vi "DAE Simple Pendulum Simulation.vi"() -> ()   [LabVIEW 2023]
doc: "This example demonstrates how to use the <B>DAE Radau 5th Order VI</B> to simulate the movement of a simple pendulum, which is modeled by a differential algebraic equation. In this example, the model is implemented by a cluster of formula strings and variable strings."
uses:
  <vilib>/gmath/dae.llb/Radau5_Parameters.ctl
  <vilib>/Analysis/1siggen.llb/Ramp Pattern by Samples.vi
  <vilib>/gmath/dae.llb/DAE Radau 5th Order (Formula).vi
  <vilib>/gmath/NI_DAE.lvlib
  <vilib>/gmath/NI_Gmath.lvlib
  <vilib>/Analysis/NI_AALBase.lvlib
panel:
  in  "Initial Position":dbl(slide)=0.8016949152542373 min=0.4 max=1.0 step=0.01 scale=0.4..1.0 scale format="%#_2g"
  out "pendulum":picture
  out "Simple Pendulum Simulation":picture
  # "Overview: This example demonstrates how to use the DAE Radau 5th Order VI to simulate the movement of a simple pendulum, which is modeled by a differential algebraic equation.\nRequirements: LabVIEW Full Development System\nInstructions: \n1. Run the VI.\n2. Change the Initial Position and run the VI again to see how the simple pendulum swings with different initial positions."
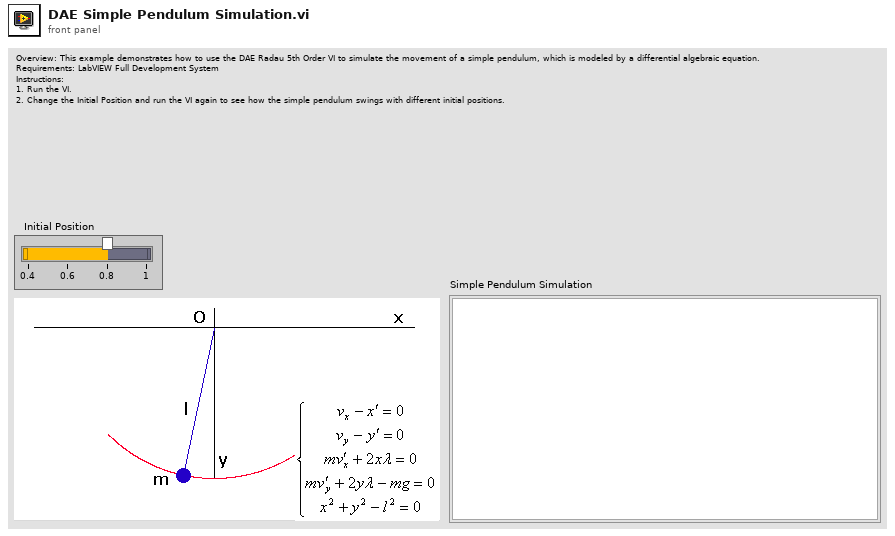
[diagram p1: front panel]
types:
  T1 = typedef "NI_DAE.lvlib/Radau5_Parameters.ctl" = cluster{"initial time":dbl, "final time":dbl, "Absolute Tolerance":dbl[], "Relative Tolerance":dbl[], "minimum time step":dbl, "maximum time step":dbl, "initial time step":dbl}
  T2 = cluster{"F(X,X',t)":string[], "X":string[], "X'":string[], "time":string}
  T3 = cluster{"Width":u16, "Style":enum32{"Solid", "Dash", "Dot", "DashDot", "DashDotDot"}}
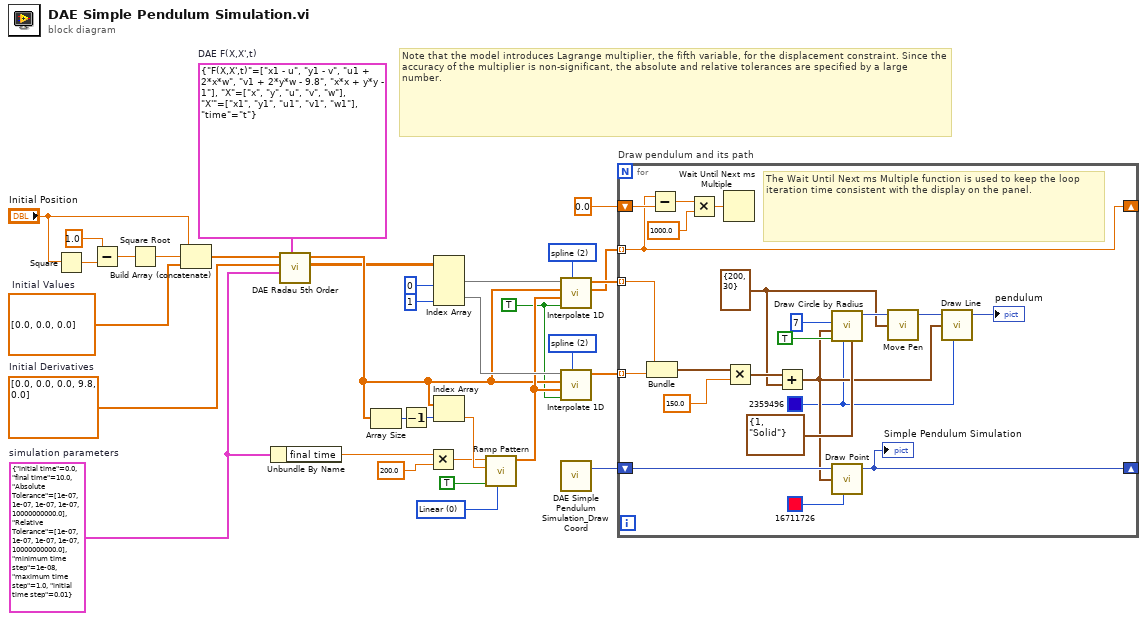
[diagram p0: block diagram]
diagram:
  w10 = T1 {"initial time"=0.0, "final time"=10.0, "Absolute Tolerance"=[1e-07, 1e-07, 1e-07, 1e-07, 10000000000.0], "Relative Tolerance"=[1e-07, 1e-07, 1e-07, 1e-07, 10000000000.0], "minimum time step"=1e-08, "maximum time step"=1.0, "initial time step"=0.01}  # simulation parameters
  w4 = dbl[] [0.0, 0.0, 0.0]  # Initial Values
  w8 = TRUE ("X is monotonic")
  w31 = 2 items=["nearest", "linear", "spline", "cubic Hermite", "Lagrange"] ("method")
  w25 = 2 items=["nearest", "linear", "spline", "cubic Hermite", "Lagrange"] ("method")
  w19 = u16 0 items=["Linear", "Logarithmic"] ("type")
  w32 = dbl[] [0.0, 0.0, 0.0, 9.8, 0.0]  # Initial Derivatives
  w33 = T2 {"F(X,X',t)"=["x1 - u", "y1 - v", "u1 + 2*x*w", "v1 + 2*y*w - 9.8", "x*x + y*y - 1"], "X"=["x", "y", "u", "v", "w"], "X'"=["x1", "y1", "u1", "v1", "w1"], "time"="t"}  # DAE F(X,X',t)
  # "Note that the model introduces Lagrange multiplier, the fifth variable, for the displacement constraint. Since the accuracy of the multiplier is non-significant, the absolute and relative tolerances are specified by a large number."
  n1 = Square(x="Initial Position") -> (x^2=w7:dbl)
  n2 = Subtract(x=1.0, y=w7) -> (x-y=w5:dbl)
  n3 = Square Root(x=w5) -> (sqrt(x)=w1:dbl)
  n4 = Build Array (concatenate)("Initial Position", w1, w4) -> (w3:dbl[])
  n5 = Unbundle By Name(w10) -> ("final time"=w9:dbl)
  n6 = call-poly <vilib>:"DAE Radau 5th Order.vi"("DAE F(X,X',t)"=w33, "simulation parameters"=w10, "Initial Derivatives"=w32, "Initial Values"=w3) -> ("X Values"=w13:dbl[][], "Times"=w14:dbl[])  [unwired: 4 in, 2 out]
  n7 = Array Size(array=w14) -> (size(s)=w27:i32)
  n8 = Decrement(x=w27) -> (x-1=w26:i32)
  n9 = Multiply(x=w9, y=200.0 ("samples")) -> (x*y=w11:dbl)
  n10 = Index Array(array=w13, index (col) #1=0 ("disabled index (col)"), index (col) #2=1 ("index (col)")) -> (element #1=w21:dbl[], element #2=w30:dbl[])  [unwired: 2 in]
  n11 = Index Array(array=w14, index=w26) -> (element=w28:dbl)
  n12 = call-poly <vilib>:"Ramp Pattern.vi"("type"=w19, "exclude end?"=TRUE, "end"=w28, "samples"=w11) -> ("Ramp Pattern"=w23:dbl[])  [unwired: 6 in, 1 out]
  n13 = call <vilib>:"Interpolate 1D.vi"("method"=w25, "X is monotonic"=w8, "xi"=w23, "X"=w14, "Y"=w21) -> ("xi used"=w20:dbl[], "yi"=w22:dbl[])  [unwired: 1 in, 4 out]
  n14 = call <vilib>:"Interpolate 1D.vi"("method"=w31, "X is monotonic"=w8, "xi"=w23, "X"=w14, "Y"=w30) -> ("yi"=w24:dbl[])  [unwired: 1 in, 5 out]
  n15 = call "DAE Simple Pendulum Simulation_Draw Coord.vi"() -> ("picture out"=w16:picture)  [unwired: 3 in]
  n16 = for "Draw pendulum and its path" {
    tunnel: w20 -> [w36] mode=indexing
    tunnel: w22 -> [w55] mode=indexing
    tunnel: w24 -> [w37] mode=indexing
    shift-right: [w43] -> _
    shift-left: w16 -> [w45]
    shift-right: [w36] -> _
    shift-left: 0.0 -> [w39]
    w41 = u32 2359496 ("color(black)")
    w47 = cluster{i16, i16} {200, 30} ("y")
    # "The Wait Until Next ms Multiple function is used to keep the loop iteration time consistent with the display on the panel."
    n17 = Bundle("Numeric"=w55, "Numeric"=w37) -> (w54:cluster{"Numeric":dbl, "Numeric":dbl})  [unwired: 1 out]
    n18 = Subtract(x=w36, y=w39) -> (x-y=w38:dbl)
    n19 = Multiply(x=w38, y=1000.0) -> (x*y=w34:dbl)
    n20 = Wait Until Next ms Multiple(millisecond multiple=w34) -> ()  [unwired: 1 out]
    n21 = Multiply(x=w54, y=150.0) -> (x*y=w52:cluster{"Numeric":dbl, "Numeric":dbl})
    n22 = Add(x=w52, y=w47) -> (x+y=w44:cluster{dbl, dbl})
    n23 = call <vilib>:"Draw Circle by Radius.vi"("pen"=T3 {"Width"=1, "Style"=enum."Solid"}, "color(black)"=w41, "fill?(F)"=TRUE, "pixel center"=w44, "radius"=i16 7) -> ("new picture"=w49:picture)  [unwired: 3 in, 3 out]
    n24 = call <vilib>:"Draw Point.vi"("picture"=w45, "point(x,y)"=w44, "color(black)"=u32 16711726) -> ("new picture"=w43:picture)  [unwired: 1 in, 5 out]
    "Simple Pendulum Simulation" <- w43
    n25 = call <vilib>:"Move Pen.vi"("new position"=w47, "picture"=w49) -> ("new picture"=w46:picture)  [unwired: 1 in, 2 out]
    n26 = call <vilib>:"Draw Line.vi"("picture"=w46, "end point"=w44, "color(black)"=w41) -> ("new picture"=→"pendulum":picture)  [unwired: 2 in, 4 out]
  }
